vi "XML429_Board_GetBoardConfig.vi"(0 "ConfigHandle in":refnum<k20>, 11 "Error in":errorcluster) -> (4 "ConfigHandle out":refnum<k20>, 6 "BoardConfig":refnum<k20>, 15 "Error out":errorcluster)   [LabVIEW 2016]
doc: "XML429_Board_GetBoardConfig"
uses:
  <vilib>/Utility/error.llb/Error Cluster From Error Code.vi
  <vilib>/ErrorRing/Error Ring.xnode
  <vilib>/xml/NI_XML.lvlib
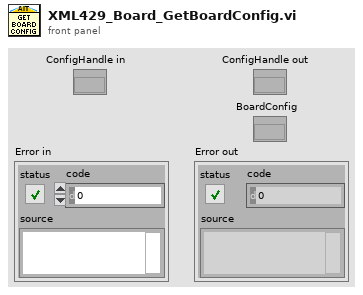
[diagram p1: front panel]
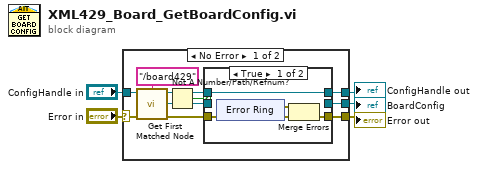
[diagram p0: block diagram]
diagram:
  n1 = case shown="No Error" "Error in" {
    selector: "Error in" -> [w15 w28]
    tunnel: [w11 w28] -> w4
    tunnel: "ConfigHandle in" -> [w14 w27]
    tunnel: [w9 w27] -> w1
    tunnel: [w6 _] -> w2
    frame No Error {
      n2 = call <vilib>:"Get First Matched Node.vi"("error in (no error)"=w15, "XPath expression"="/board429", "node in"=w14) -> ("error out"=w12:errorcluster, "node result"=w7:refnum<k20>, "node out"=w10:refnum<k20>)  [unwired: 6 in]
      n3 = Not A Number/Path/Refnum?(number/path/refnum=w7) -> (NaN/Path/Refnum?=w8:bool)
      n4 = case shown="True" w8 {
        tunnel: [w16 w26] -> w11
        tunnel: w12 -> [w18 w26]
        tunnel: [w19 w25] -> w9
        tunnel: w10 -> [w19 w25]
        tunnel: [_ w24] -> w6
        tunnel: w7 -> [_ w24]
        frame True {
          n5 = xnode "Error Ring"() -> ("error out"=w17:errorcluster)
          n6 = Merge Errors(w18, w17) -> (w16:errorcluster)
        }
        frame False, Default {
        }
      }
    }
    frame Error {
    }
  }
  "Error out" <- w4
  "BoardConfig" <- w2
  "ConfigHandle out" <- w1
